vi "Swerve Debug.vi"(10 "Controller":dbl) -> ()   [LabVIEW 2017]
uses:
  <vilib>/Rock Robotics/WPI/ThirdParty/Phoenix-LabVIEW/Motor Controller/Controls/CTRE_Phoenix_MotorControl_ControlMode.ctl
  Public/Documents/Cross The Road Electronics/Phoenix-LabVIEW/Motor Controller/Get/CTRE_Phoenix_MotorController_GetPulseWidthAll.vi
  Robot Global Data.vi
panel:
  in  "BR Spin 2":bool
  in  "FR Spin 2":bool
  in  "BL Spin 2":bool
  in  "FL Spin 2":bool
  in  "Enable Offset":bool
  in  "Global Position":dbl step=1024.0
  in  "Global Position":bool
  in  "Drive via Controler Yaxis":bool
  in  "BR Drive":bool
  in  "BL Drive":bool
  in  "FR Drive":bool
  in  "FL Drive":bool
  in  "BR Spin":bool
  in  "BL Spin":bool
  in  "FR Spin":bool
  in  "FL Spin":bool
  out "BR CPosition":dbl
  out "BL CPosition":dbl
  out "FR CPosition":dbl
  out "FL CPosition":dbl
  in  "BR Position":dbl step=1024.0
  in  "BL Position":dbl step=1024.0
  in  "FR Position":dbl step=1024.0
  in  "FL Position":dbl step=1024.0
  in  "Drive Motor":dbl step=0.05
  # "Enable Output"
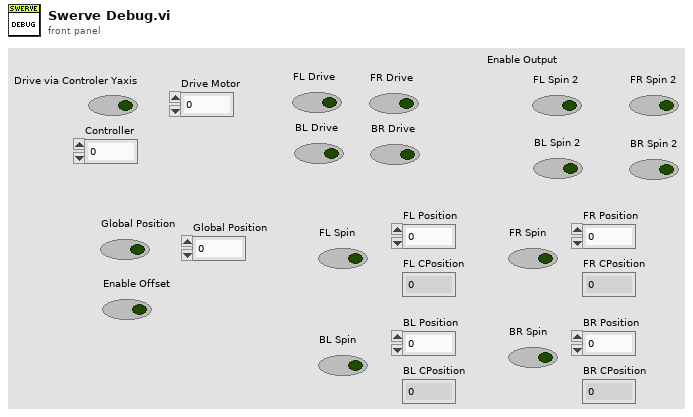
[diagram p1: front panel]
types:
  T1 = typedef "WPI_MotorControlDeviceRef.ctl" = cluster{"DeviceStatus":errorcluster, "Type":T2, "PWM":cluster{"PWM Channel":T3, "DeadBand":T4}, "CAN":cluster{"Device Number":u8, "SetOutput VI Ref":variant, "GetOutput VI Ref":variant, "Enable VI Ref":variant, "Disable VI Ref":variant, "Data":variant}, "Invert":bool, "DIO PWM":cluster{"PWM \"Enable\" Channel":T3, "DIOChannel":T5, "PWM Rate":dbl}}
  T2 = typedef "WPI_MotorControlType.ctl" = enum16{"PWM", "CAN", "DIO PWM"}
  T3 = typedef "FPGA_DIOPWMChannel.ctl" = enum8{"PWM 0", "PWM 1", "PWM 2", "PWM 3", "PWM 4", "PWM 5", "PWM 6", "PWM 7", "PWM 8", "PWM 9", "PWM MXP 0", "PWM MXP 1", "PWM MXP 2", "PWM MXP 3", "PWM MXP 4", "PWM MXP 5", "PWM MXP 6", "PWM MXP 7", "PWM MXP 8", "PWM MXP 9", "Invalid"}
  T4 = typedef "WPI_PWMDeadband.ctl" = cluster{"Name":string, "maxPositivePwm":i32, "minPositivePwm":i32, "centerPwm":i32, "maxNegativePwm":i32, "minNegativePwm":i32, "angularRange":u16}
  T5 = typedef "FPGA_DIOChannel.ctl" = enum8{"DIO 0", "DIO 1", "DIO 2", "DIO 3", "DIO 4", "DIO 5", "DIO 6", "DIO 7", "DIO 8", "DIO 9", "DIO MXP 0", "DIO MXP 1", "DIO MXP 2", "DIO MXP 3", "DIO MXP 4", "DIO MXP 5", "DIO MXP 6", "DIO MXP 7", "DIO MXP 8", "DIO MXP 9", "DIO MXP 10", "DIO MXP 11", "DIO MXP 12", "DIO MXP 13", "DIO MXP 14", "DIO MXP 15", "SPI Port CS1", "SPI Port CS2", "SPI Port CS3", "SPI Port MISO", "SPI Port MOSI", "Invalid"}
  T6 = typedef "CTRE_Phoenix_MotorControl_ControlMode.ctl" = u16
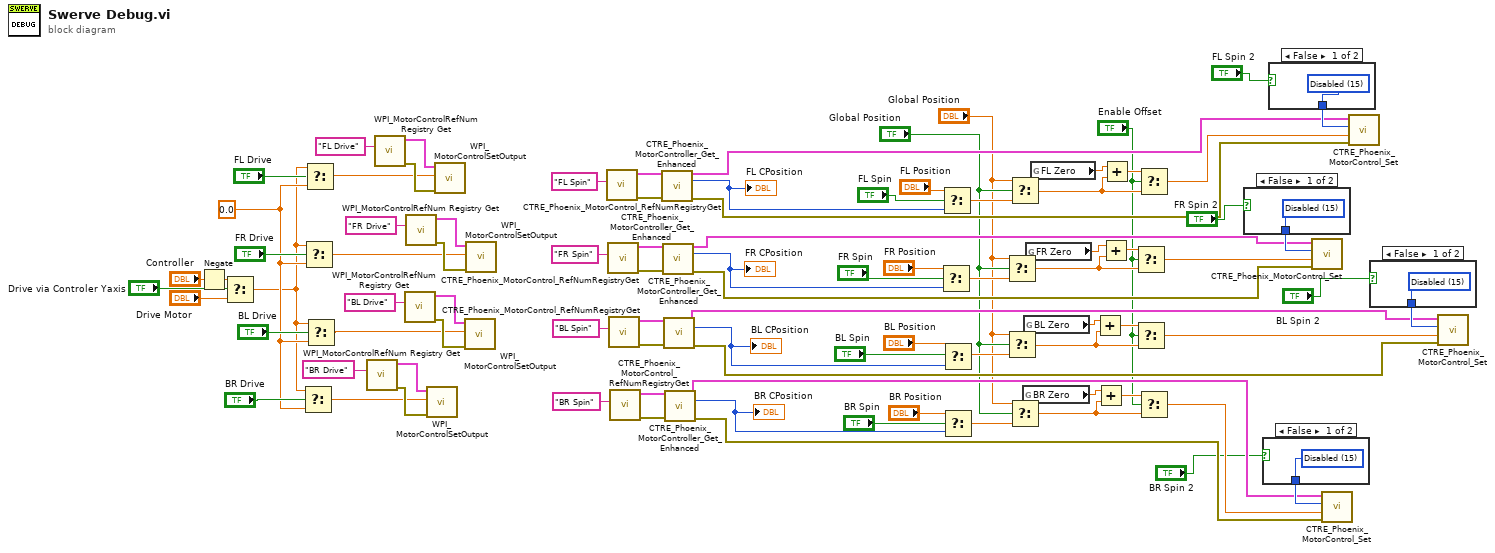
[diagram p0: block diagram]
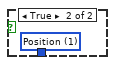
[diagram p2: hidden frame]
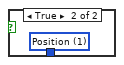
[diagram p3: hidden frame]
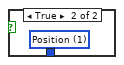
[diagram p4: hidden frame]
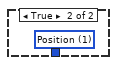
[diagram p5: hidden frame]
diagram:
  w69 = 0.0 ("f")
  n1 = Negate(x="Controller") -> (-x=w5:dbl)
  n2 = Select(t=w5, s="Drive via Controler Yaxis", f="Drive Motor") -> (s? t:f=w65:dbl)
  n3 = Select(t=w65, s="BR Drive", f=w69) -> (s? t:f=w74:dbl)
  n4 = Select(t=w65, s="FR Drive", f=w69) -> (s? t:f=w76:dbl)
  n5 = Select(t=w65, s="FL Drive", f=w69) -> (s? t:f=w78:dbl)
  n6 = Select(t=w65, s="BL Drive", f=w69) -> (s? t:f=w75:dbl)
  n7 = call <vilib>:"WPI_MotorControlRefNum Registry Get.vi"("refnum name"="BR Drive") -> ("error out"=w79:errorcluster, "MotorControlDevRef"=w80:T1)  [unwired: 9 in]
  n8 = call <vilib>:"WPI_MotorControlRefNum Registry Get.vi"("refnum name"="FL Drive") -> ("error out"=w87:errorcluster, "MotorControlDevRef"=w89:T1)  [unwired: 9 in]
  n9 = call <vilib>:"WPI_MotorControlRefNum Registry Get.vi"("refnum name"="BL Drive") -> ("error out"=w81:errorcluster, "MotorControlDevRef"=w83:T1)  [unwired: 9 in]
  n10 = call <vilib>:"WPI_MotorControlRefNum Registry Get.vi"("refnum name"="FR Drive") -> ("error out"=w84:errorcluster, "MotorControlDevRef"=w86:T1)  [unwired: 9 in]
  n11 = call <vilib>:"WPI_MotorControlSetOutput.vi"("error in (no error)"=w79, "Output"=w74, "MotorControlDevRef"=w80) -> ()  [unwired: 6 in, 3 out]
  n12 = call <vilib>:"WPI_MotorControlSetOutput.vi"("error in (no error)"=w87, "Output"=w78, "MotorControlDevRef"=w89) -> ()  [unwired: 6 in, 3 out]
  n13 = call <vilib>:"WPI_MotorControlSetOutput.vi"("error in (no error)"=w81, "Output"=w75, "MotorControlDevRef"=w83) -> ()  [unwired: 6 in, 3 out]
  n14 = call <vilib>:"WPI_MotorControlSetOutput.vi"("error in (no error)"=w84, "Output"=w76, "MotorControlDevRef"=w86) -> ()  [unwired: 6 in, 3 out]
  n15 = call "CTRE_Phoenix_MotorControl_RefNumRegistryGet.vi"("refnum name"="FL Spin") -> ("error out"=w55:errorcluster, "PhoenixMotorControlDevRef"=w56:T1)  [unwired: 9 in]
  n16 = call "CTRE_Phoenix_MotorControl_RefNumRegistryGet.vi"("refnum name"="FR Spin") -> ("error out"=w46:errorcluster, "PhoenixMotorControlDevRef"=w47:T1)  [unwired: 9 in]
  n17 = call "CTRE_Phoenix_MotorControl_RefNumRegistryGet.vi"("refnum name"="BL Spin") -> ("error out"=w43:errorcluster, "PhoenixMotorControlDevRef"=w44:T1)  [unwired: 9 in]
  n18 = call "CTRE_Phoenix_MotorControl_RefNumRegistryGet.vi"("refnum name"="BR Spin") -> ("error out"=w40:errorcluster, "PhoenixMotorControlDevRef"=w41:T1)  [unwired: 9 in]
  n19 = call-poly "CTRE_Phoenix_MotorController_Get_Enhanced.vi"("PhoenixMotorControlDevRef"=w56, "error in"=w55) -> ("PhoenixMotorControlDevRef"=w34:T1, "Pulse Width Position"=w38:i32, "error out"=w27:errorcluster)  [unwired: 8 in, 3 out]
  "FL CPosition" <- w38
  n20 = call-poly "CTRE_Phoenix_MotorController_Get_Enhanced.vi"("PhoenixMotorControlDevRef"=w47, "error in"=w46) -> ("PhoenixMotorControlDevRef"=w33:T1, "Pulse Width Position"=w37:i32, "error out"=w28:errorcluster)  [unwired: 8 in, 3 out]
  "FR CPosition" <- w37
  n21 = call-poly "CTRE_Phoenix_MotorController_Get_Enhanced.vi"("PhoenixMotorControlDevRef"=w44, "error in"=w43) -> ("PhoenixMotorControlDevRef"=w32:T1, "Pulse Width Position"=w36:i32, "error out"=w29:errorcluster)  [unwired: 8 in, 3 out]
  "BL CPosition" <- w36
  n22 = call-poly "CTRE_Phoenix_MotorController_Get_Enhanced.vi"("PhoenixMotorControlDevRef"=w41, "error in"=w40) -> ("PhoenixMotorControlDevRef"=w31:T1, "Pulse Width Position"=w35:i32, "error out"=w30:errorcluster)  [unwired: 8 in, 3 out]
  "BR CPosition" <- w35
  n23 = Select(t="FR Position", s="FR Spin", f=w37) -> (s? t:f=w48:dbl)
  n24 = Select(t="FL Position", s="FL Spin", f=w38) -> (s? t:f=w52:dbl)
  n25 = Select(t="BL Position", s="BL Spin", f=w36) -> (s? t:f=w26:dbl)
  n26 = Select(t="BR Position", s="BR Spin", f=w35) -> (s? t:f=w25:dbl)
  n27 = Select(t="Global Position", s="Global Position", f=w48) -> (s? t:f=w12:dbl)
  n28 = Select(t="Global Position", s="Global Position", f=w26) -> (s? t:f=w13:dbl)
  n29 = Select(t="Global Position", s="Global Position", f=w52) -> (s? t:f=w11:dbl)
  n30 = Select(t="Global Position", s="Global Position", f=w25) -> (s? t:f=w14:dbl)
  n31 = global read "Robot Global Data.vi" "BR Zero"() -> (w6:dbl)
  n32 = global read "Robot Global Data.vi" "BL Zero"() -> (w7:dbl)
  n33 = global read "Robot Global Data.vi" "FR Zero"() -> (w8:dbl)
  n34 = global read "Robot Global Data.vi" "FL Zero"() -> (w9:dbl)
  n35 = Add(x=w7, y=w13) -> (x+y=w16:dbl)
  n36 = Add(x=w6, y=w14) -> (x+y=w15:dbl)
  n37 = Add(x=w8, y=w12) -> (x+y=w17:dbl)
  n38 = Add(x=w9, y=w11) -> (x+y=w18:dbl)
  n39 = Select(t=w17, s="Enable Offset", f=w12) -> (s? t:f=w20:dbl)
  n40 = Select(t=w16, s="Enable Offset", f=w13) -> (s? t:f=w22:dbl)
  n41 = Select(t=w18, s="Enable Offset", f=w11) -> (s? t:f=w19:dbl)
  n42 = Select(t=w15, s="Enable Offset", f=w14) -> (s? t:f=w21:dbl)
  n43 = case shown="False" "FR Spin 2" {
    tunnel: [w90 w91] -> w51
    frame False {
      w90 = T6 15 items=["PercentOutput"=0, "Position"=1, "Velocity"=2, "Current"=3, "Follower"=5, "MotionProfile"=6, "MotionMagic"=7, "MotionMagicArc"=8, "MotionProfileArc"=10, "Disabled"=15] ("Control Mode")
    }
    frame True {
      w91 = T6 1 items=["PercentOutput"=0, "Position"=1, "Velocity"=2, "Current"=3, "Follower"=5, "MotionProfile"=6, "MotionMagic"=7, "MotionMagicArc"=8, "MotionProfileArc"=10, "Disabled"=15] ("Control Mode")
    }
  }
  n44 = case shown="False" "BR Spin 2" {
    tunnel: [w92 w93] -> w49
    frame False {
      w92 = T6 15 items=["PercentOutput"=0, "Position"=1, "Velocity"=2, "Current"=3, "Follower"=5, "MotionProfile"=6, "MotionMagic"=7, "MotionMagicArc"=8, "MotionProfileArc"=10, "Disabled"=15] ("Control Mode")
    }
    frame True {
      w93 = T6 1 items=["PercentOutput"=0, "Position"=1, "Velocity"=2, "Current"=3, "Follower"=5, "MotionProfile"=6, "MotionMagic"=7, "MotionMagicArc"=8, "MotionProfileArc"=10, "Disabled"=15] ("Control Mode")
    }
  }
  n45 = case shown="False" "FL Spin 2" {
    tunnel: [w94 w95] -> w53
    frame False {
      w94 = T6 15 items=["PercentOutput"=0, "Position"=1, "Velocity"=2, "Current"=3, "Follower"=5, "MotionProfile"=6, "MotionMagic"=7, "MotionMagicArc"=8, "MotionProfileArc"=10, "Disabled"=15] ("Control Mode")
    }
    frame True {
      w95 = T6 1 items=["PercentOutput"=0, "Position"=1, "Velocity"=2, "Current"=3, "Follower"=5, "MotionProfile"=6, "MotionMagic"=7, "MotionMagicArc"=8, "MotionProfileArc"=10, "Disabled"=15] ("Control Mode")
    }
  }
  n46 = call <vilib>:"CTRE_Phoenix_MotorControl_Set.vi"("error in (no error)"=w28, "Output"=w20, "Control Mode"=w51, "PhoenixMotorControlDevRef"=w33) -> ()  [unwired: 6 in, 2 out]
  n47 = call <vilib>:"CTRE_Phoenix_MotorControl_Set.vi"("error in (no error)"=w30, "Output"=w21, "Control Mode"=w49, "PhoenixMotorControlDevRef"=w31) -> ()  [unwired: 6 in, 2 out]
  n48 = call <vilib>:"CTRE_Phoenix_MotorControl_Set.vi"("error in (no error)"=w27, "Output"=w19, "Control Mode"=w53, "PhoenixMotorControlDevRef"=w34) -> ()  [unwired: 6 in, 2 out]
  n49 = case shown="False" "BL Spin 2" {
    tunnel: [w96 w97] -> w50
    frame False {
      w96 = T6 15 items=["PercentOutput"=0, "Position"=1, "Velocity"=2, "Current"=3, "Follower"=5, "MotionProfile"=6, "MotionMagic"=7, "MotionMagicArc"=8, "MotionProfileArc"=10, "Disabled"=15] ("Control Mode")
    }
    frame True {
      w97 = T6 1 items=["PercentOutput"=0, "Position"=1, "Velocity"=2, "Current"=3, "Follower"=5, "MotionProfile"=6, "MotionMagic"=7, "MotionMagicArc"=8, "MotionProfileArc"=10, "Disabled"=15] ("Control Mode")
    }
  }
  n50 = call <vilib>:"CTRE_Phoenix_MotorControl_Set.vi"("error in (no error)"=w29, "Output"=w22, "Control Mode"=w50, "PhoenixMotorControlDevRef"=w32) -> ()  [unwired: 6 in, 2 out]
